vi "Main Process Case.vi"(8 "error in (no error)":errorcluster, 10 "CurrentAction":string, 11 "Main Process Class in":refnum<class "MPC_AutoInspection.lvclass">) -> (0 "error out":errorcluster, 1 "KeepCase":bool, 3 "Main Process Class out":refnum<class "MPC_AutoInspection.lvclass">)   [LabVIEW 2019, in "MPC_AutoInspection.lvclass"]
uses:
  MPC_AutoInspection.lvclass
  Ctrl/Auto Inspection Station Name2.ctl
  Ctrl/Auto Inspection Data Name.ctl
  Ctrl/ModbusCmd.ctl
  Ctrl/123.ctl
  9bf7879c-bf60-4f24-9d05-9736aede328f.vi
  <vilib>/JDP Science/JSONtext/JSON text to Variant.vi
  LLB/Commonly VI/Main Glb.vi
  Global/Process Global.vi
  LLB/Commonly VI.lvlib
  Ctrl/Project Flow ChoiceS1.ctl
  Ctrl/ProjectAct Step.ctl
panel:
  out "step content 2":string[](array[string])
  in  "$Read Project Recipe":path=path "C:/Users/MyUser/Desktop/S2_Project.txt"
  out "DataOut":string
  out "Boolean 2":bool=TRUE
  out "Boolean":bool=TRUE
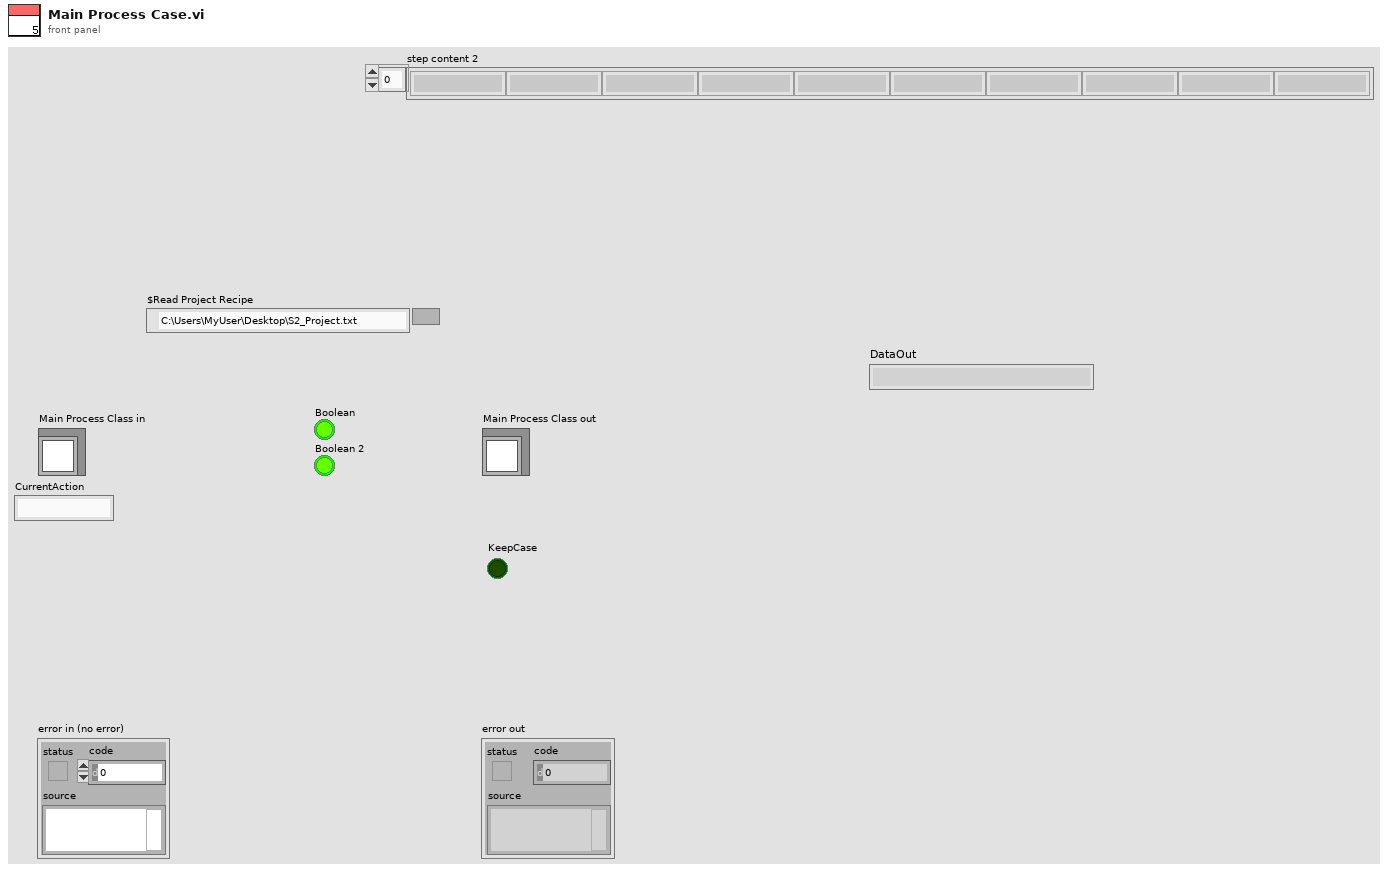
[diagram p1: front panel]
types:
  T1 = cluster{"starting address":u16, "number of inputs":u16, "Sat Coils":bool[], "Holding Registers":u16[]}
  T2 = typedef "ModbusCmd.ctl" = enum16{"Connect", "Disconnect", "Init", "Fetch Basic Objects", "Fetch Input Refisters", "Fetch Discrete Inputs", "Set Coils", "Set Holding Registers", "Write Single Holding", "Exit"}
  T3 = typedef "Auto Inspection Station Name2.ctl" = enum16{"S1Barcode", "S2Measure", "S3Measure", "S4Measure", "S5Measure", "S11_LaserCheck", "S8_Vision AI"}
  T4 = typedef "Auto Inspection Data Name.ctl" = enum16{"LocalRun", "ItemSN(TimeCode)", "CurrentAction", "Error", "Data", "OKNG", "電壓值", "電壓值判斷", "電流值", "電流值判斷", "Laser1 Data", "Laser2 Data", "Laser OKNG", "StationNO"}
  T5 = typedef "123.ctl" = enum16{"Initial", "Write", "Read"}
  T6 = cluster{"AutoRunFlg":refnum<vi>, "Action Finish Flg":refnum<vi>, "Remaining Action":refnum<vi>, "Btn_AutoRun":refnum<vi>, "Manual Flg":refnum<vi>, "Sub Process Error":refnum<vi>}
  T7 = enum16{"Initial", "load", "read", "write", "write sn", "save"}
  T8 = typedef "ProjectAct Step.ctl" = enum16{"ProjectName", "Name", "Initial", "Reset", "Format", "Program1", "Program2", "Scan"}
  T9 = typedef "Project Flow ChoiceS1.ctl" = enum16{"Chk Modbus Connect", "Chk Start", "Chk Project", "Initial", "Reset", "Format", "Program", "Scan"}
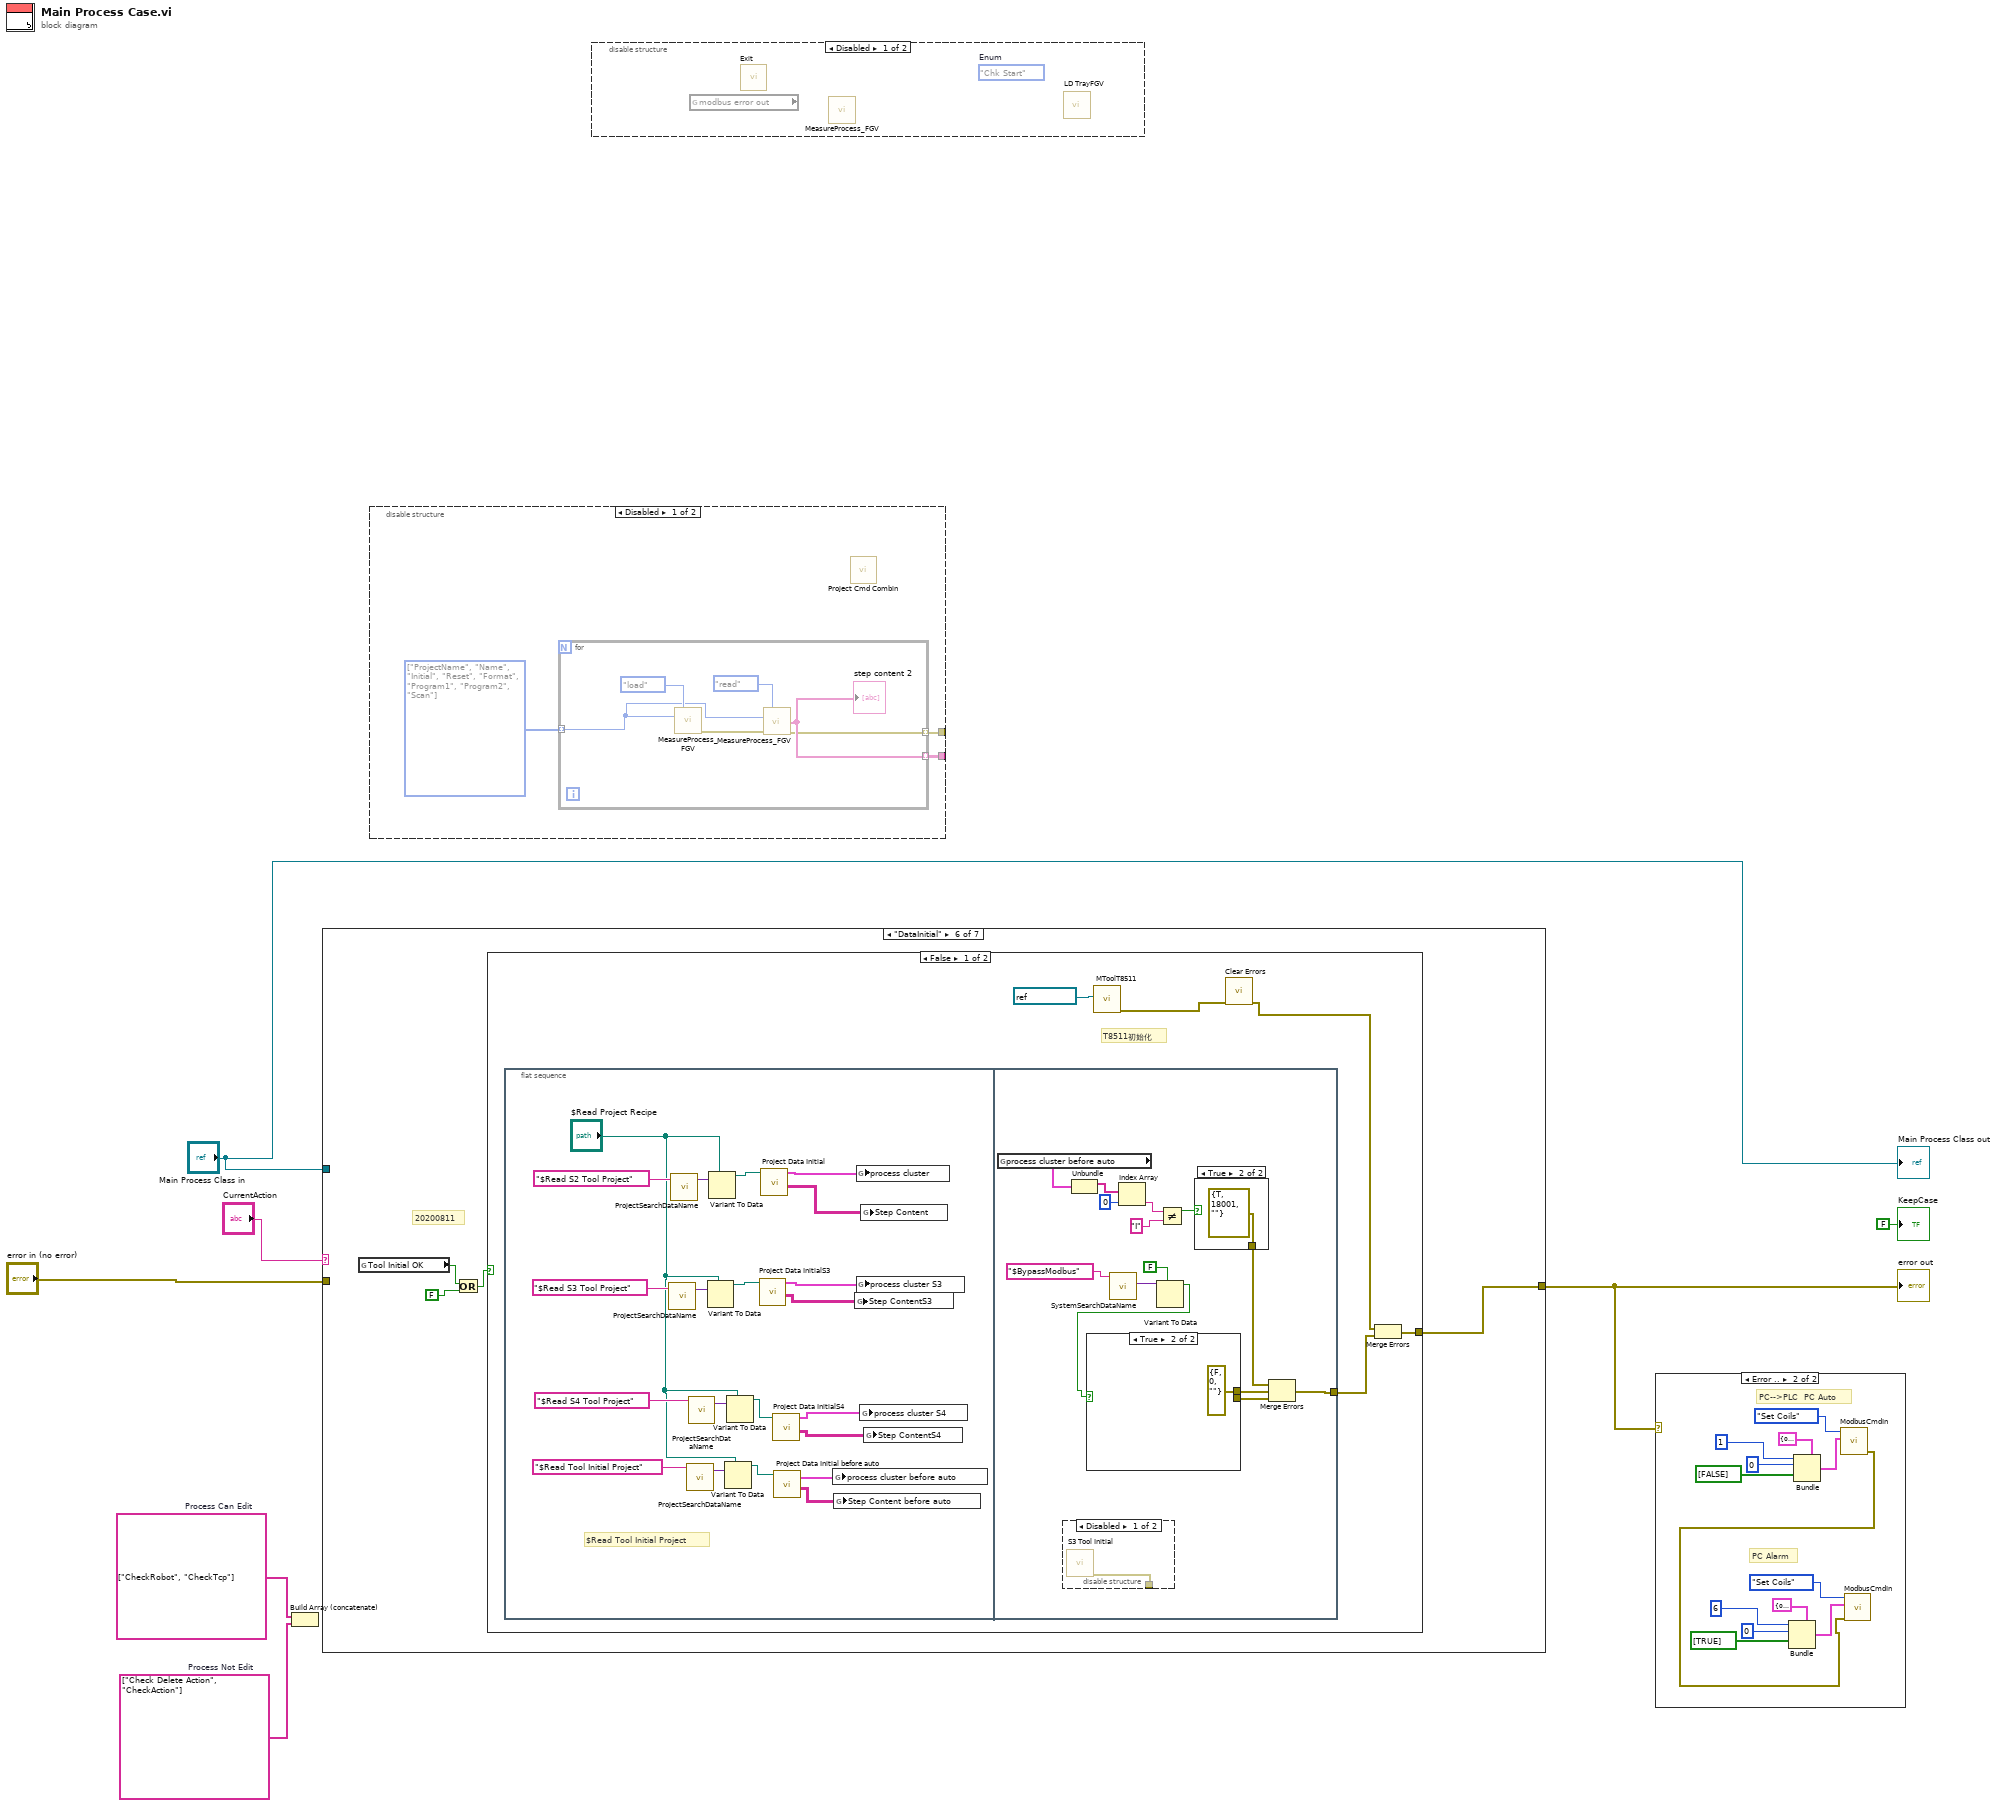
[diagram p0: block diagram]
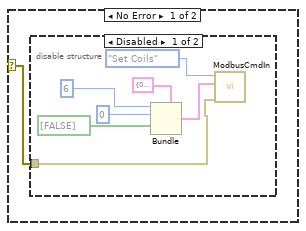
[diagram p3: hidden frame]
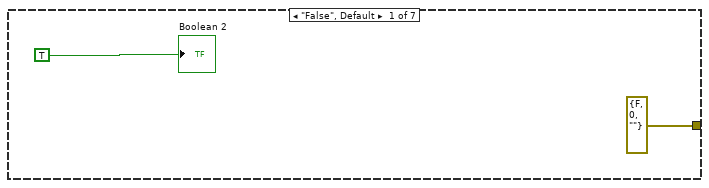
[diagram p6: hidden frame]
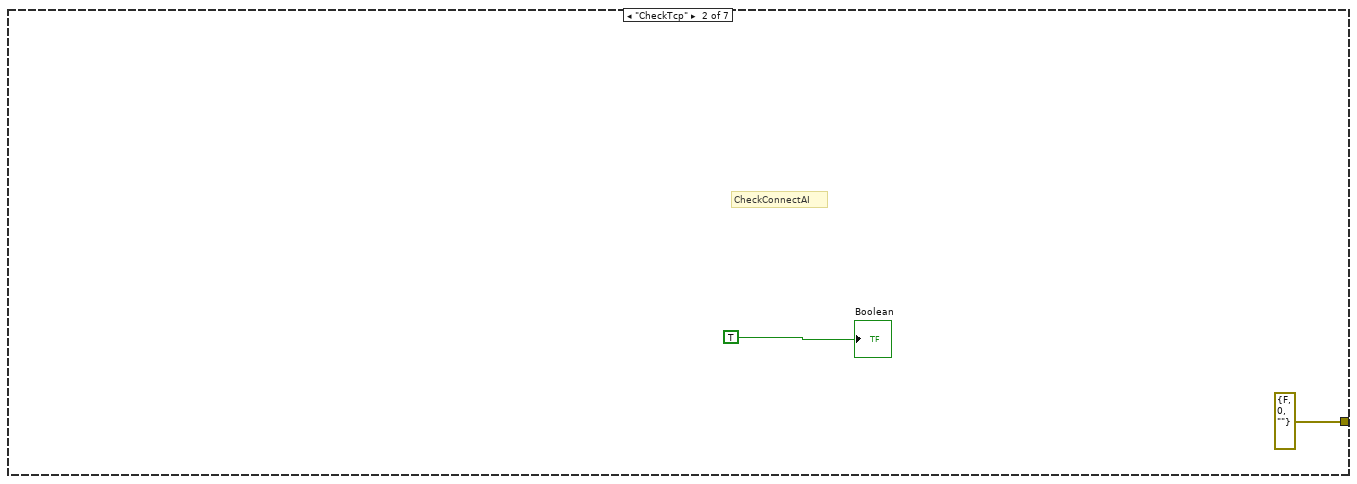
[diagram p7: hidden frame]
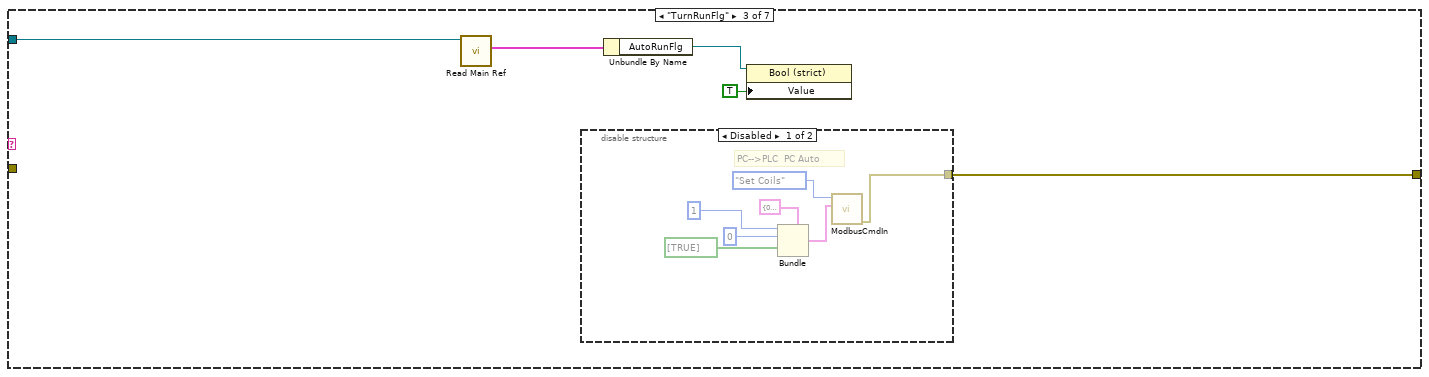
[diagram p8: hidden frame]
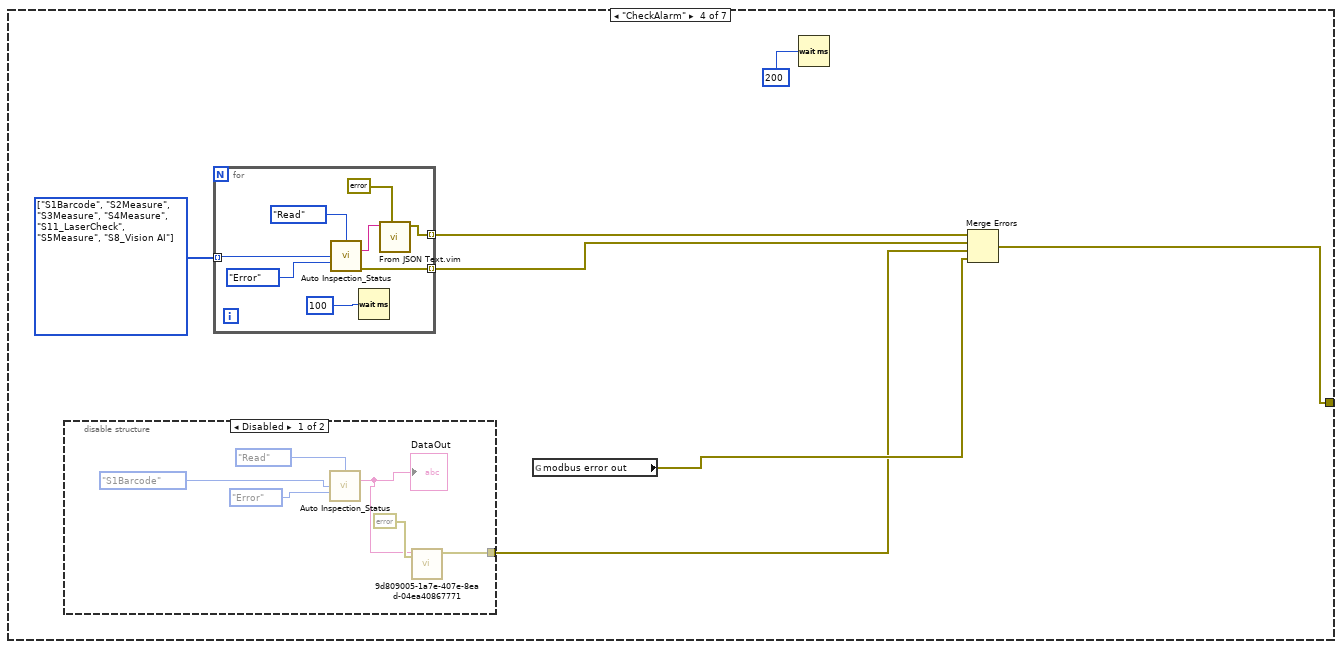
[diagram p10: hidden frame]
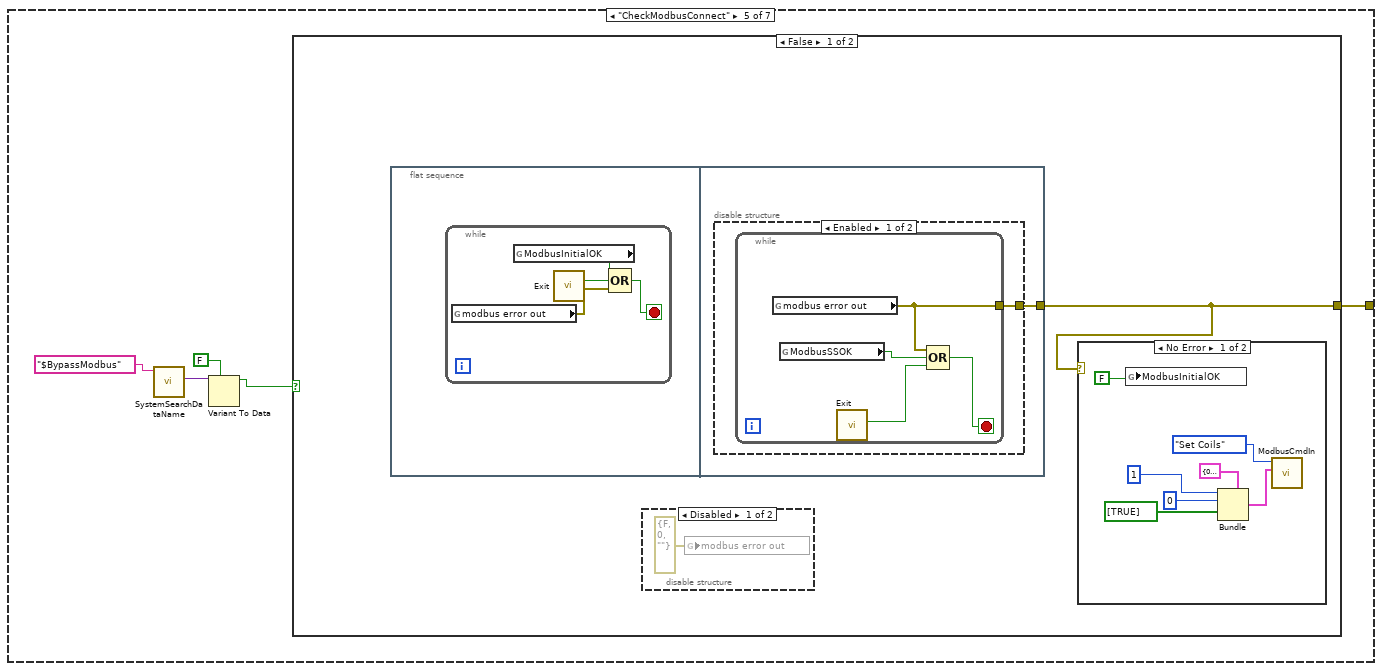
[diagram p12: hidden frame]
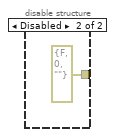
[diagram p15: hidden frame]
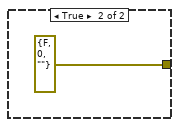
[diagram p16: hidden frame]
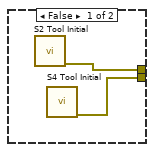
[diagram p17: hidden frame]
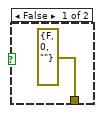
[diagram p19: hidden frame]
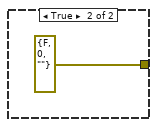
[diagram p20: hidden frame]
diagram:
  w5 = string[] ["Check Delete Action", "CheckAction"]  # Process Not Edit
  w6 = string[] ["CheckRobot", "CheckTcp"]  # Process Can Edit
  n1 = Build Array (concatenate)(w6, w5) -> ()  [unwired: 1 out]
  n2 = case shown="\"DataInitial\"" "CurrentAction" {
    tunnel: "error in (no error)" -> [_ _ _ _ _ _ _]
    tunnel: "Main Process Class in" -> [_ _ w16 _ _ _ _]
    tunnel: [errorcluster {"status"=FALSE, "code"=0, "source"=""} ("modbus error out") errorcluster {"status"=FALSE, "code"=0, "source"=""} ("modbus error out") w12 w28 w49 w74 w129] -> w2
    frame "False", Default {
      "Boolean 2" <- TRUE
    }
    frame "CheckTcp" {
      # "CheckConnectAI"
      "Boolean" <- TRUE ("Boolean")
    }
    frame "TurnRunFlg" {
      n3 = call-dynamic "Read Main Ref.vi"("Main Process Class in"=w16) -> ("Main Ref"=w15:T6)  [unwired: 8 in, 2 out]
      n4 = disable-structure shown="Disabled" {
        disable-tunnel: [w17 _] -> w12
        frame Disabled {
          # "PC-->PLC  PC Auto"
          n5 = Bundle(cluster=T1 {"starting address"=0, "number of inputs"=0, "Sat Coils"=[], "Holding Registers"=[]} ("data"), "starting address"=1, "number of inputs"=u16 0, "Sat Coils"=bool[] [TRUE]) -> (w23:T1)  [unwired: 1 in]
          n6 = call "ModbusCmdIn.vi"("data"=w23, "Enum"=ModbusCmd."Set Coils") -> ("error out"=w17:errorcluster)  [unwired: 9 in]
        }
        frame Enabled {
        }
      }
      n7 = Unbundle By Name(w15) -> ("AutoRunFlg"=w14:refnum<vi>)
      n8 = property class="Bool (strict)"(reference=w14, "Value"=TRUE) -> ()  [unwired: 1 in, 2 out]
    }
    frame "CheckAlarm" {
      w27 = T3[] [enum."S1Barcode", enum."S2Measure", enum."S3Measure", enum."S4Measure", enum."S11_LaserCheck", enum."S5Measure", enum."S8_Vision AI"] items=["S1Barcode", "S2Measure", "S3Measure", "S4Measure", "S5Measure", "S11_LaserCheck", "S8_Vision AI"]
      n9 = disable-structure shown="Disabled" {
        disable-tunnel: [w31 _] -> w25
        frame Disabled {
          n10 = call "Auto Inspection_Status.vi"("Action"=enum16{"Initial", "Write", "Read"}."Read", "Station"=Auto_Inspection_Station_Name2."S1Barcode", "Data"=Auto_Inspection_Data_Name."Error") -> ("DataOut"=w32:string)  [unwired: 10 in, 2 out]
          "DataOut" <- w32
          n11 = call "9d809005-1a7e-407e-8ead-04ea40867771.vi"("Data Type and Default Value"=errorcluster {"status"=FALSE, "code"=0, "source"=""} ("error constant"), "JSON"=w32) -> ("Data out"=w31:errorcluster)  [unwired: 8 in, 1 out]
        }
        frame Enabled {
        }
      }
      n12 = for {
        tunnel: w27 -> [w43] mode=indexing
        tunnel: [w42] -> w26 mode=indexing
        tunnel: [w37] -> w24 mode=indexing
        n13 = call "Auto Inspection_Status.vi"("Action"=enum16{"Initial", "Write", "Read"}."Read", "Station"=w43, "Data"=Auto_Inspection_Data_Name."Error") -> ("DataOut"=w39:string, "error out"=w42:errorcluster)  [unwired: 10 in, 1 out]
        n14 = Wait (ms)(milliseconds to wait=100) -> ()  [unwired: 1 out]
        n15 = call "From JSON Text.vim"("Data Type and Default Value"=errorcluster {"status"=FALSE, "code"=0, "source"=""} ("error constant"), "JSON"=w39) -> ("Data out"=w37:errorcluster)  [unwired: 8 in, 1 out]
      }
      n16 = global read "Main Glb.vi" "modbus error out"() -> (w29:errorcluster)
      n17 = Wait (ms)(milliseconds to wait=u32 200) -> ()  [unwired: 1 out]
      n18 = Merge Errors(w24, w26, w25, w29) -> (w28:errorcluster)
    }
    frame "CheckModbusConnect" {
      n19 = call "SystemSearchDataName.vi"("element"="$BypassModbus") -> ("variant"=w46:variant)  [unwired: 8 in, 2 out]
      n20 = Variant To Data(type=FALSE, Variant=w46) -> (data=w45:bool)  [unwired: 1 in, 1 out]
      n21 = case shown="False" w45 {
        tunnel: [w50 errorcluster {"status"=FALSE, "code"=0, "source"=""} ("modbus error out")] -> w49
        frame False {
          n22 = flat-sequence {
            tunnel: [w63] -> w50
            frame #0 {
              n23 = while {
                stop <- w62 stop-if-true
                n24 = global read "Main Glb.vi" "modbus error out"() -> (w59:errorcluster)
                n25 = global read "Main Glb.vi" "ModbusInitialOK"() -> (w61:bool)
                n26 = call "Exit.vi"() -> ("ExitOut"=w60:bool)  [unwired: 11 in]
                n27 = Compound Arithmetic op=OR(w61, w60, w59) -> (w62:bool)
              }
            }
            frame #1 {
              n28 = disable-structure shown="Enabled" {
                disable-tunnel: [w64 errorcluster {"status"=FALSE, "code"=0, "source"=""} ("modbus error out")] -> w63
                frame Enabled {
                  n29 = while {
                    tunnel: [w68] -> w64
                    stop <- w67 stop-if-true
                    n30 = global read "Main Glb.vi" "modbus error out"() -> (w68:errorcluster)
                    n31 = global read "Main Glb.vi" "ModbusSSOK"() -> (w66:bool)
                    n32 = call "Exit.vi"() -> ("ExitOut"=w65:bool)  [unwired: 11 in]
                    n33 = Compound Arithmetic op=OR(w68, w66, w65) -> (w67:bool)
                  }
                }
                frame Disabled {
                }
              }
            }
          }
          n34 = disable-structure shown="Disabled" {
            frame Disabled {
              n35 = global write "Main Glb.vi" "modbus error out"(errorcluster {"status"=FALSE, "code"=0, "source"=""} ("modbus error out")) -> ()
            }
            frame Enabled {
            }
          }
          n36 = case shown="No Error" w50 {
            frame No Error {
              n37 = global write "Main Glb.vi" "ModbusInitialOK"(FALSE) -> ()
              n38 = Bundle(cluster=T1 {"starting address"=0, "number of inputs"=0, "Sat Coils"=[], "Holding Registers"=[]} ("data"), "starting address"=1, "number of inputs"=u16 0, "Sat Coils"=bool[] [TRUE]) -> (w56:T1)  [unwired: 1 in]
              n39 = call "ModbusCmdIn.vi"("data"=w56, "Enum"=ModbusCmd."Set Coils") -> ()  [unwired: 9 in, 1 out]
            }
            frame Error {
            }
          }
        }
        frame True {
        }
      }
    }
    frame "DataInitial" {
      # "20200811"
      n40 = global read "Process Global.vi" "Tool Initial OK"() -> (w73:bool)
      n41 = Or(x=w73, y=FALSE) -> (x .or. y?=w71:bool)
      n42 = case shown="False" w71 {
        tunnel: [w78 errorcluster {"status"=FALSE, "code"=0, "source"=""} ("error IO")] -> w74
        frame False {
          # "T8511初始化"
          n43 = flat-sequence {
            tunnel: [w114] -> w77
            frame #0 {
              # "$Read Tool Initial Project"
              n44 = call "ProjectSearchDataName.vi"("element"="$Read S3 Tool Project") -> ("variant"=w89:variant)  [unwired: 7 in, 3 out]
              n45 = call "ProjectSearchDataName.vi"("element"="$Read S2 Tool Project") -> ("variant"=w94:variant)  [unwired: 7 in, 3 out]
              n46 = call "ProjectSearchDataName.vi"("element"="$Read Tool Initial Project") -> ("variant"=w82:variant)  [unwired: 7 in, 3 out]
              n47 = call "ProjectSearchDataName.vi"("element"="$Read S4 Tool Project") -> ("variant"=w86:variant)  [unwired: 7 in, 3 out]
              n48 = Variant To Data(type="$Read Project Recipe", Variant=w89) -> (data=w91:path)  [unwired: 1 in, 1 out]
              n49 = Variant To Data(type="$Read Project Recipe", Variant=w94) -> (data=w92:path)  [unwired: 1 in, 1 out]
              n50 = Variant To Data(type="$Read Project Recipe", Variant=w82) -> (data=w81:path)  [unwired: 1 in, 1 out]
              n51 = Variant To Data(type="$Read Project Recipe", Variant=w86) -> (data=w84:path)  [unwired: 1 in, 1 out]
              n52 = call "Project Data InitialS3.vi"("configuration file path"=w91) -> ("Step Content"=w88:string[][], "process cluster"=w87:cluster{string[], i32[]})  [unwired: 8 in, 1 out]
              n53 = call "Project Data Initial.vi"("configuration file path"=w92) -> ("Step Content"=w99:string[][], "process cluster"=w100:cluster{string[], i32[]})  [unwired: 7 in, 2 out]
              n54 = call "Project Data InitialS4.vi"("configuration file path"=w84) -> ("Step Content"=w98:string[][], "process cluster"=w97:cluster{string[], i32[]})  [unwired: 8 in, 1 out]
              n55 = call "Project Data Initial before auto.vi"("configuration file path"=w81) -> ("Step Content"=w95:string[][], "process cluster"=w96:cluster{string[], i32[]})  [unwired: 7 in, 2 out]
              n56 = global write "Process Global.vi" "process cluster before auto"(w96) -> ()
              n57 = global write "Process Global.vi" "Step Content before auto"(w95) -> ()
              n58 = global write "Process Global.vi" "Step ContentS3"(w88) -> ()
              n59 = global write "Process Global.vi" "process cluster"(w100) -> ()
              n60 = global write "Process Global.vi" "process cluster S3"(w87) -> ()
              n61 = global write "Process Global.vi" "process cluster S4"(w97) -> ()
              n62 = global write "Process Global.vi" "Step Content"(w99) -> ()
              n63 = global write "Process Global.vi" "Step ContentS4"(w98) -> ()
            }
            frame #1 {
              n64 = global read "Process Global.vi" "process cluster before auto"() -> (w113:cluster{string[], i32[]})
              n65 = disable-structure shown="Disabled" {
                disable-tunnel: [w118 _] -> _
                frame Disabled {
                  n66 = call "S3 Tool Initial.vi"() -> ("error constant"=w118:errorcluster)  [unwired: 11 in]
                }
                frame Enabled {
                }
              }
              n67 = Unbundle(w113) -> (w112:string[])  [unwired: 1 out]
              n68 = call "SystemSearchDataName.vi"("element"="$BypassModbus") -> ("variant"=w104:variant)  [unwired: 8 in, 2 out]
              n69 = Index Array(array=w112, index=0) -> (element=w109:string)
              n70 = Variant To Data(type=FALSE, Variant=w104) -> (data=w101:bool)  [unwired: 1 in, 1 out]
              n71 = case shown="True" w101 {
                tunnel: [w116 errorcluster {"status"=FALSE, "code"=0, "source"=""} ("error constant")] -> w106
                tunnel: [w115 _] -> w105
                frame False {
                  n72 = call "S2 Tool Initial.vi"() -> ("error constant"=w116:errorcluster)  [unwired: 10 in, 1 out]
                  n73 = call "S4 Tool Initial.vi"() -> ("error constant"=w115:errorcluster)  [unwired: 10 in, 1 out]
                }
                frame True {
                }
              }
              n74 = Not Equal?(x=w109, y="I") -> (x != y?=w108:bool)
              n75 = case shown="True" w108 {
                tunnel: [errorcluster {"status"=FALSE, "code"=0, "source"=""} ("error constant") errorcluster {"status"=TRUE, "code"=18001, "source"=""} ("error constant")] -> w107
                frame False {
                }
                frame True {
                }
              }
              n76 = Merge Errors(w107, w106, w105) -> (w114:errorcluster)
            }
          }
          n77 = call "MToolT8511.vi"("VISA resource name"=refnum<visa-resource-name> "COM11") -> ("error out"=w76:errorcluster)  [unwired: 9 in, 1 out]
          n78 = call <vilib>:"Clear Errors.vi"("error in (no error)"=w76) -> ("error out"=w75:errorcluster)  [unwired: 5 in, 1 out]
          n79 = Merge Errors(w75, w77) -> (w78:errorcluster)
        }
        frame True {
        }
      }
    }
    frame "ToolInitial" {
      # "20200811"
      n80 = call "Station Initial Status.vi"("Insert"=0, "Enum"=123."Read") -> ("Read"=w126:bool)  [unwired: 8 in, 1 out]
      n81 = Equal?(x=w126, y=TRUE) -> (x = y?=w124:bool)
      n82 = Or(x=w124, y=FALSE) -> (x .or. y?=w122:bool)
      n83 = case shown="False" w122 {
        tunnel: [w132 errorcluster {"status"=FALSE, "code"=0, "source"=""} ("error IO")] -> w129
        frame False {
          # "Initial Cmd In"
          n84 = disable-structure shown="Disabled" {
            disable-tunnel: [w140 _] -> w131
            disable-tunnel: [w139 _] -> w130
            frame Disabled {
              n85 = for {
                N: 3 -> [_]
                tunnel: [w144] -> _
                tunnel: [w143] -> w139
                stop <- w147 stop-if-true
                w146 = u16 0 items=["INITIAL", "RESET", "FORMAT", "PROGRAM1", "PROGRAM2", "FSKSCAN", "ASKSCAN"] ("action")
                # "S3測試站Initial"
                n86 = call "Tool RS232 testS3.vi"("VISA resource name"=refnum<visa-resource-name> "COM3", "action"=w146) -> ("error out"=w143:errorcluster, "receive string"=w144:string)  [unwired: 8 in]
                n87 = Unbundle By Name(w143) -> ("status"=w148:bool)
                n88 = Not(x=w148) -> (.not. x?=w147:bool)
              }
              n89 = for {
                N: 3 -> [_]
                tunnel: [w150] -> _
                tunnel: [w149] -> w140
                stop <- w153 stop-if-true
                w152 = u16 0 items=["INITIAL", "RESET", "FORMAT", "PROGRAM1", "PROGRAM2", "FSKSCAN", "ASKSCAN"] ("action")
                # "S2測試站Initial"
                n90 = call "Tool RS232 testS2.vi"("VISA resource name"=refnum<visa-resource-name> "COM3", "action"=w152) -> ("error out"=w149:errorcluster, "receive string"=w150:string)  [unwired: 8 in]
                n91 = Unbundle By Name(w149) -> ("status"=w154:bool)
                n92 = Not(x=w154) -> (.not. x?=w153:bool)
              }
            }
            frame Enabled {
            }
          }
          n93 = disable-structure shown="Disabled" {
            frame Disabled {
              n94 = Select(t=TRUE ("Status"), s=TRUE, f=FALSE) -> (s? t:f=w134:bool)
              n95 = call "Station Initial Status.vi"("Status"=w134, "Insert"=0, "Enum"=123."Write") -> ()  [unwired: 7 in, 2 out]
            }
            frame Enabled {
            }
          }
          n96 = Merge Errors(w131, w130) -> (w132:errorcluster)
        }
        frame True {
        }
      }
    }
  }
  "error out" <- w2
  n97 = disable-structure shown="Disabled" {
    disable-tunnel: [w158 _] -> _
    disable-tunnel: [w156 _] -> _
    frame Disabled {
      w157 = T8[] [enum."ProjectName", enum."Name", enum."Initial", enum."Reset", enum."Format", enum."Program1", enum."Program2", enum."Scan"] items=["ProjectName", "Name", "Initial", "Reset", "Format", "Program1", "Program2", "Scan"]
      n98 = for {
        tunnel: w157 -> [w161] mode=indexing
        tunnel: [w160] -> w158 mode=indexing
        tunnel: [w159] -> w156 mode=indexing
        n99 = call "MeasureProcess_FGV.vi"("action"=T7."load", "ProjectAct step"=w161) -> ("error out"=w162:errorcluster)  [unwired: 9 in, 4 out]
        n100 = call "MeasureProcess_FGV.vi"("action"=T7."read", "ProjectAct step"=w161, "error in"=w162) -> ("step content"=w160:string[], "error out"=w159:errorcluster)  [unwired: 8 in, 3 out]
        "step content 2" <- w160
      }
      n101 = call "Project Cmd Combin.vi"() -> ()  [unwired: 9 in, 3 out]
    }
    frame Enabled {
    }
  }
  n102 = disable-structure shown="Disabled" {
    frame Disabled {
      (unwired) Project_Flow_ChoiceS1."Chk Start"  # Enum
      n103 = global read "Main Glb.vi" "modbus error out"() -> ()  [unwired: 1 out]
      n104 = call "Exit.vi"() -> ()  [unwired: 11 in, 1 out]
      n105 = call "MeasureProcess_FGV.vi"() -> ()  [unwired: 11 in, 5 out]
      n106 = call "LD TrayFGV.vi"() -> ()  [unwired: 10 in, 2 out]
    }
    frame Enabled {
    }
  }
  n107 = case shown="Error .." w2 {
    selector: w2 -> [w165 _]
    frame No Error {
      n108 = disable-structure shown="Disabled" {
        disable-tunnel: w165 -> [w166 _]
        frame Disabled {
          n109 = Bundle(cluster=T1 {"starting address"=0, "number of inputs"=0, "Sat Coils"=[], "Holding Registers"=[]} ("data"), "starting address"=6, "number of inputs"=u16 0, "Sat Coils"=bool[] [FALSE]) -> (w172:T1)  [unwired: 1 in]
          n110 = call "ModbusCmdIn.vi"("error in (no error)"=w166, "data"=w172, "Enum"=ModbusCmd."Set Coils") -> ()  [unwired: 8 in, 1 out]
        }
        frame Enabled {
        }
      }
    }
    frame Error {
      # "PC Alarm"
      # "PC-->PLC  PC Auto"
      n111 = Bundle(cluster=T1 {"starting address"=0, "number of inputs"=0, "Sat Coils"=[], "Holding Registers"=[]} ("data"), "starting address"=6, "number of inputs"=u16 0, "Sat Coils"=bool[] [TRUE]) -> (w179:T1)  [unwired: 1 in]
      n112 = Bundle(cluster=T1 {"starting address"=0, "number of inputs"=0, "Sat Coils"=[], "Holding Registers"=[]} ("data"), "starting address"=1, "number of inputs"=u16 0, "Sat Coils"=bool[] [FALSE]) -> (w185:T1)  [unwired: 1 in]
      n113 = call "ModbusCmdIn.vi"("data"=w185, "Enum"=ModbusCmd."Set Coils") -> ("error out"=w173:errorcluster)  [unwired: 9 in]
      n114 = call "ModbusCmdIn.vi"("error in (no error)"=w173, "data"=w179, "Enum"=ModbusCmd."Set Coils") -> ()  [unwired: 8 in, 1 out]
    }
  }
  "Main Process Class out" <- "Main Process Class in"
  "KeepCase" <- FALSE ("KeepCase")
